vi "Pre-Actor.vi"(8 "error in":errorcluster, 11 "DAQ970 in":refnum<class "DAQ970.lvclass">) -> (0 "error out":errorcluster, 3 "DAQ970 out":refnum<class "DAQ970.lvclass">)   [LabVIEW 2019, in "DAQ970.lvlib" / "DAQ970.lvclass"]
doc: "This override VI is to provide the means for children classes to perform application specific post launch initialization functions that must be performed *prior* to calling the actor. \n\n***DO NOT USE THE CHECK FOR FAULT ROUTINE HERE***"
uses:
  Library/DAQ970.lvclass
  Library/DAQ970.lvclass/DAQ970.ctl
  builds/Instruments/Instruments.lvlibp/Library/Instruments.lvclass
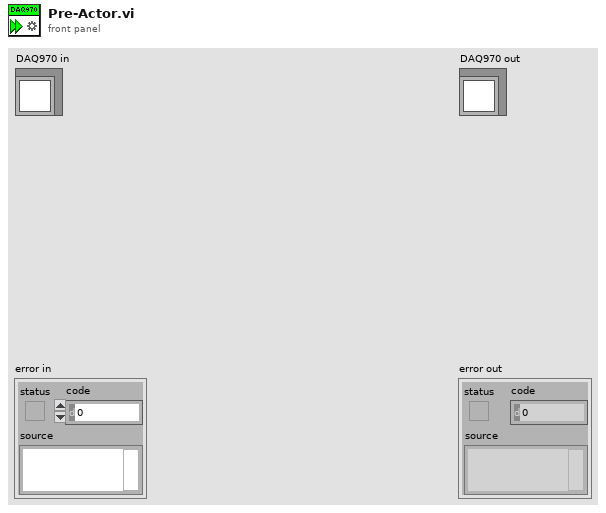
[diagram p1: front panel]
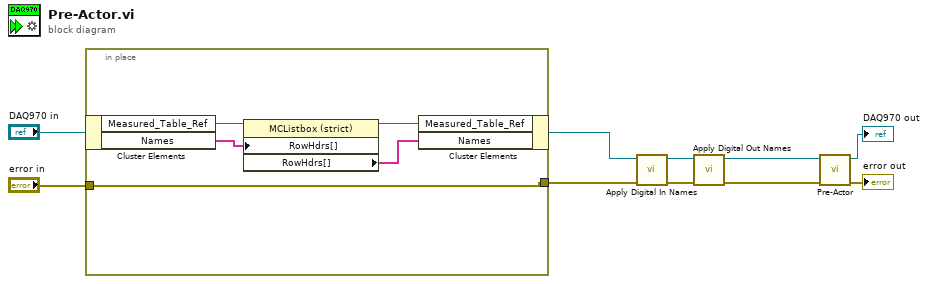
[diagram p0: block diagram]
diagram:
  n1 = in-place {
    in-place-border: [w11] -> w3
    in-place-border: "error in" -> [w11]
    n2 = in-place-cluster #1("DAQ970 in") -> ("Measured_Table_Ref"=w15:refnum<vi>, "Names"=w13:string[])
    n3 = property class="MCListbox (strict)"(reference=w15, "RowHdrs[]"=w13) -> (reference out=w14:refnum<vi>, "RowHdrs[]"=w12:string[])  [unwired: 1 in, 1 out]
    n4 = in-place-cluster #1("Measured_Table_Ref"=w14, "Names"=w12) -> (w4:refnum<class "DAQ970.lvclass">)
  }
  n5 = call "Apply Digital In Names.vi"("error in (no error)"=w3, "DAQ970 in"=w4) -> ("error out"=w5:errorcluster, "DAQ970 out"=w6:refnum<class "DAQ970.lvclass">)  [unwired: 8 in]
  n6 = call "Apply Digital Out Names.vi"("error in (no error)"=w5, "DAQ970 in"=w6) -> ("error out"=w1:errorcluster, "DAQ970 out"=w2:refnum<class "DAQ970.lvclass">)  [unwired: 8 in]
  n7 = call-parent "Pre-Actor.vi"("error in (no error)"=w1, "Instruments in"=w2) -> ("error out"=→"error out":errorcluster, "Instruments out"=→"DAQ970 out":refnum<class "DAQ970.lvclass">)  [unwired: 8 in]
